vi "set output trigger.vi"(8 "error in (no error)":errorcluster, 11 "DAQOrcaFlash in":refnum<class "DAQOrcaFlash.lvclass">) -> (0 "error out":errorcluster, 3 "DAQOrcaFlash out":refnum<class "DAQOrcaFlash.lvclass">)   [LabVIEW 2012, in "DAQOrcaFlash.lvclass"]
uses:
  DAQOrcaFlash.lvclass
  connector.ctl
  DAQOrcaFlash.lvclass/DAQOrcaFlash.ctl
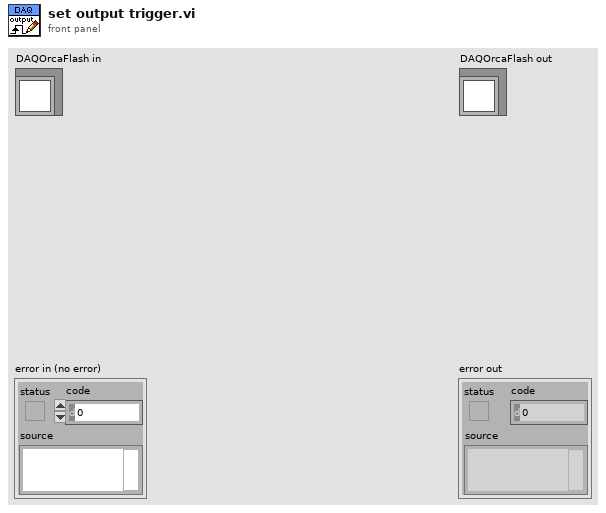
[diagram p1: front panel]
types:
  T1 = typedef "DAQOrcaFlash.lvclass/connector.ctl" = enum32{"1", "2", "3"}
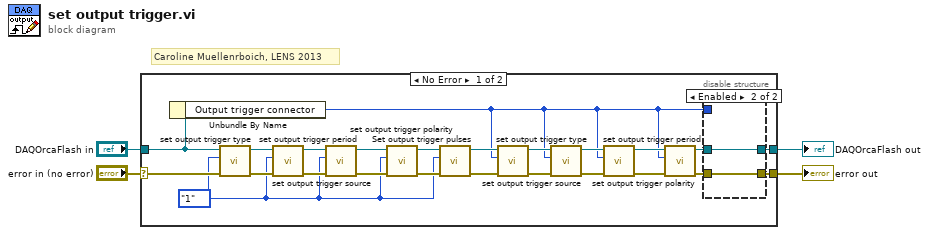
[diagram p0: block diagram]
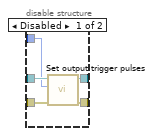
[diagram p2: hidden frame]
diagram:
  # "Caroline Muellenrboich, LENS 2013"
  n1 = case shown="No Error" "error in (no error)" {
    selector: "error in (no error)" -> [w16 w37]
    tunnel: [w5 w37] -> w4
    tunnel: [w7 w36] -> w2
    tunnel: "DAQOrcaFlash in" -> [w15 w36]
    frame No Error {
      w10 = connector."1" ("Output trigger connector")
      n2 = Unbundle By Name(w15) -> ("Output trigger connector"=w6:T1)
      n3 = call-dynamic "set output trigger type.vi"("error in (no error)"=w16, "Output trigger connector"=w10, "DAQOrcaFlash in"=w15) -> ("error out"=w20:errorcluster, "DAQOrcaFlash out"=w22:refnum<class "DAQOrcaFlash.lvclass">)  [unwired: 7 in]
      n4 = call-dynamic "set output trigger source.vi"("error in (no error)"=w20, "Output trigger connector"=w10, "DAQOrcaFlash in"=w22) -> ("error out"=w19:errorcluster, "DAQOrcaFlash out"=w21:refnum<class "DAQOrcaFlash.lvclass">)  [unwired: 7 in]
      n5 = call-dynamic "set output trigger period.vi"("error in (no error)"=w19, "Output trigger connector"=w10, "DAQOrcaFlash in"=w21) -> ("error out"=w17:errorcluster, "DAQOrcaFlash out"=w18:refnum<class "DAQOrcaFlash.lvclass">)  [unwired: 7 in]
      n6 = call-dynamic "set output trigger polarity.vi"("error in (no error)"=w17, "Output trigger connector"=w10, "DAQOrcaFlash in"=w18) -> ("error out"=w14:errorcluster, "DAQOrcaFlash out"=w12:refnum<class "DAQOrcaFlash.lvclass">)  [unwired: 7 in]
      n7 = call-dynamic "Set output trigger pulses.vi"("error in (no error)"=w14, "Output trigger connector"=w10, "DAQOrcaFlash in"=w12) -> ("error out"=w13:errorcluster, "DAQOrcaFlash out"=w11:refnum<class "DAQOrcaFlash.lvclass">)  [unwired: 7 in]
      n8 = call-dynamic "set output trigger type.vi"("error in (no error)"=w13, "Output trigger connector"=w6, "DAQOrcaFlash in"=w11) -> ("error out"=w26:errorcluster, "DAQOrcaFlash out"=w28:refnum<class "DAQOrcaFlash.lvclass">)  [unwired: 7 in]
      n9 = call-dynamic "set output trigger source.vi"("error in (no error)"=w26, "Output trigger connector"=w6, "DAQOrcaFlash in"=w28) -> ("error out"=w25:errorcluster, "DAQOrcaFlash out"=w27:refnum<class "DAQOrcaFlash.lvclass">)  [unwired: 7 in]
      n10 = call-dynamic "set output trigger period.vi"("error in (no error)"=w25, "Output trigger connector"=w6, "DAQOrcaFlash in"=w27) -> ("error out"=w23:errorcluster, "DAQOrcaFlash out"=w24:refnum<class "DAQOrcaFlash.lvclass">)  [unwired: 7 in]
      n11 = call-dynamic "set output trigger polarity.vi"("error in (no error)"=w23, "Output trigger connector"=w6, "DAQOrcaFlash in"=w24) -> ("error out"=w9:errorcluster, "DAQOrcaFlash out"=w8:refnum<class "DAQOrcaFlash.lvclass">)  [unwired: 7 in]
      n12 = disable-structure shown="Enabled" {
        disable-tunnel: w9 -> [w33 w35]
        disable-tunnel: w8 -> [w31 w34]
        disable-tunnel: [w30 w34] -> w7
        disable-tunnel: w6 -> [w29 _]
        disable-tunnel: [w32 w35] -> w5
        frame Disabled {
          n13 = call-dynamic "Set output trigger pulses.vi"("error in (no error)"=w33, "Output trigger connector"=w29, "DAQOrcaFlash in"=w31) -> ("error out"=w32:errorcluster, "DAQOrcaFlash out"=w30:refnum<class "DAQOrcaFlash.lvclass">)  [unwired: 7 in]
        }
        frame Enabled {
        }
      }
    }
    frame Error {
    }
  }
  "error out" <- w4
  "DAQOrcaFlash out" <- w2
